vi "OE2011&OE2021_Configure Auto Phase And Filter.vi"(7 "OE2011&OE2021_\nAuto Phase And Filter":T1={"Auto Phase"=FALSE, "Auto Filter"=FALSE, "Demodulator"=1} {"Demodulator" items=["Demod1"=1, "Demod2"=2, "Demod3"=3, "Demod4"=4, "Demod5"=5, "Demod6"=6, "Demod7"=7, "Demod8"=8]}, 8 "Error in (no error)":errorcluster caption="error out（no error）", 9 "Remote Mode":u16(ring) items=["USB", "RS232", "GPIB", "Ethernet"], 10 "Connection ID in":refnum<k5>, 11 "VISA resource name":refnum<visa-resource-name>) -> (0 "Error out":errorcluster caption="error out", 1 "Output String":string, 2 "Connection ID out":refnum<k5>, 3 "VISA resource  out":refnum<visa-resource-name>)   [LabVIEW 2011]
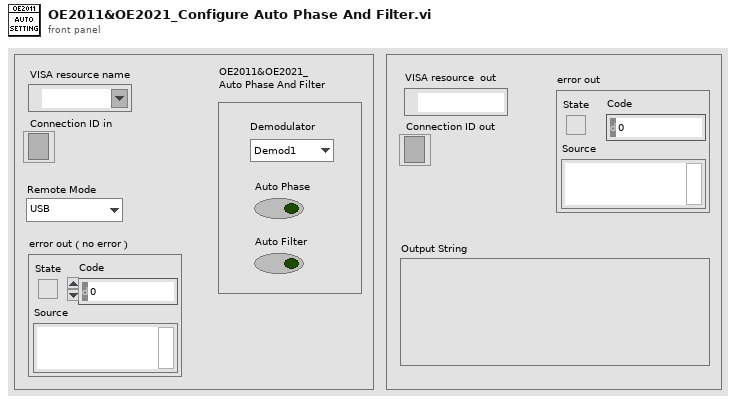
[diagram p1: front panel]
types:
  T1 = cluster{"Auto Phase":bool, "Auto Filter":bool, "Demodulator":u16}
  T2 = enum16{"ISRC", "IGND", "ICPL", "ILIN", "PHAS", "FMOD", "RSLP", "FREQ", "SWPT", "SLLM", "SULM", "SSLL", "SSLG", "STLM", "SWRM", "IRNG", "SENS", "RMOD", "OFLT", "OFSL", "SYNC", "DMOD", "HARM", "DARB", "SWVT", "SLVL", "SVLL", "SVUL", "SVSL", "SVSG", "SVTM", "SVRM", "RALL", "SNAP", "OUTP", "OAUX", "COUT", "CAUX", "COFP", "CEXP", "FPOP", "OEXP", "*IDN", "*RST", "OVLD", "INOV", "GNOV", "*PLL", "SSET", "RSET", "AGAN", "APHS", "ARSV", "ASCL", "EQCD", "EQCS", "SPED", "SRAT", "SLEN", "SSLE", "STRG", "SPRM", "STRD", "PAUS", "REST", "SPTS", "TRCA", "TEMP", "RSTU", "IHNZ", "DEQU", "SADD", "ARNG", "CSPE", "ISRCD", "IGNDD", "ICPLD", "ILIND", "PHASD", "FMODD", "RSLPD", "FREQD", "SWPTD", "SLLMD", "SULMD", "SSLLD", "SSLGD", "STLMD", "SWRMD", "SENSD", "RMODD", "OFLTD", "OFSLD", "SYNCD", "HARMD", "EQCDD", "EQCSD", "SNAPD", "OUTPD", "SWVTD", "SLVLD", "SVLLD", "SVULD", "SVSLD", "SVSGD", "SVTMD", "SVRMD", "SVDCD", "ARSVD", "AGAND", "APHSD", "ASCLD", "FPOPD", "CAUXD", "OEXPD", "SPEDD", "SRATD", "SLEND", "SSLED", "STRGD", "SPRMD", "STRDD", "PAUSD", "RESTD", "SPTSD", "TRCAD", "*IDND", "*RSTD", "INOVD", "GNOVD", "*PLLD", "SSETD", "RSETD"}
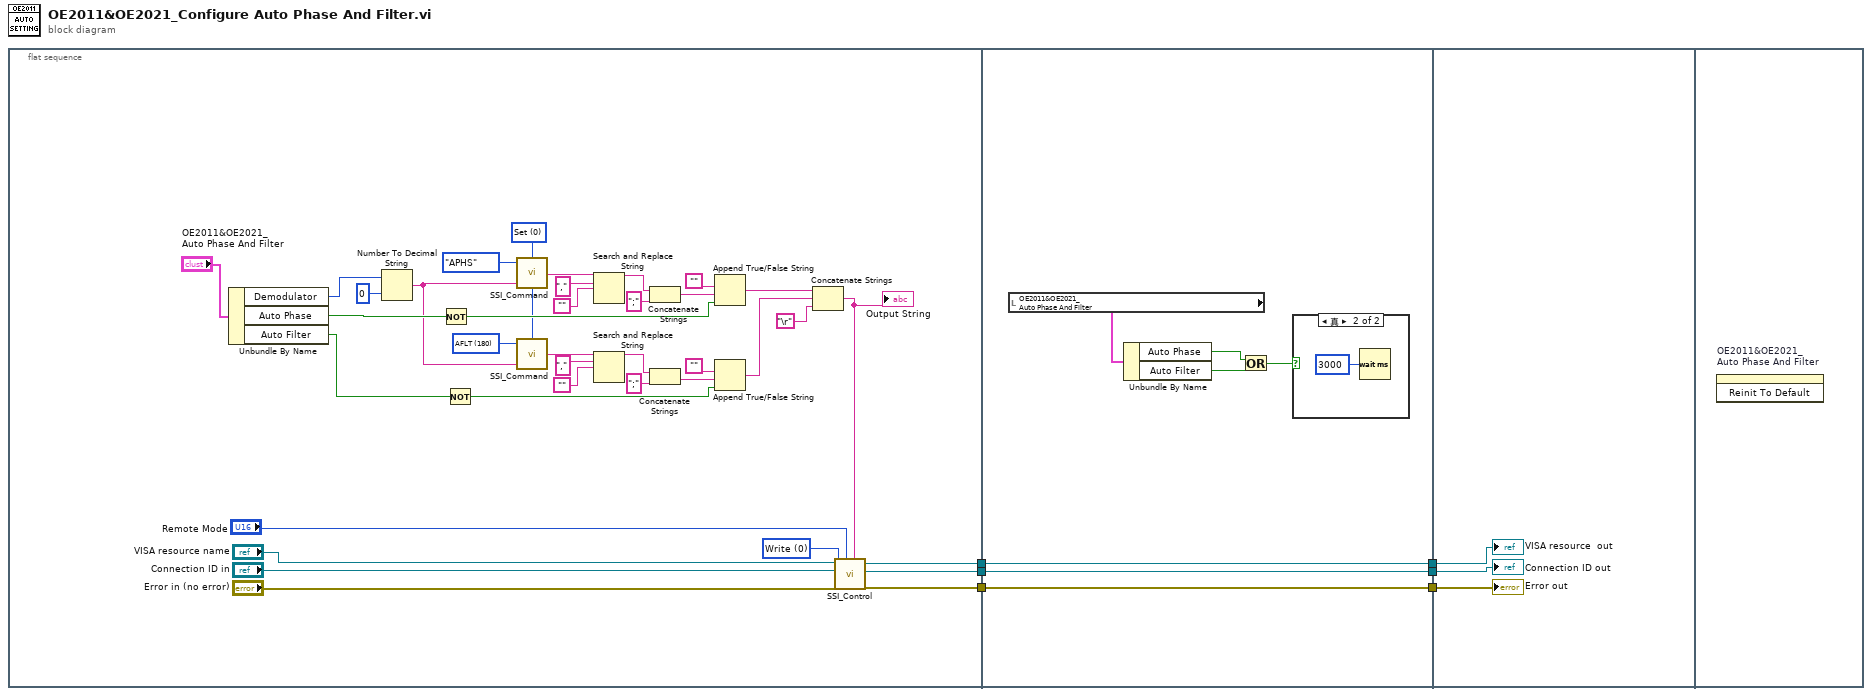
[diagram p0: block diagram]
diagram:
  n1 = flat-sequence {
    tunnel: [w39] -> w6
    tunnel: [w38] -> w5
    tunnel: [w37] -> w4
    tunnel: w6 -> [w50]
    tunnel: w5 -> [w49]
    tunnel: w4 -> [w48]
    tunnel: [w50] -> w3
    tunnel: [w49] -> w2
    tunnel: [w48] -> w1
    tunnel: w3 -> [w53]
    tunnel: w2 -> [w54]
    tunnel: w1 -> [w52]
    frame #0 {
      w13 = u16 0 items=["Set", "Query"] ("Opera")
      w18 = u16 180 items=["ISRC", "IGND", "ICPL", "ILIN", "PHAS", "FMOD", "RSLP", "FREQ", "SWPT", "SLLM", "SULM", "SSLL", "SSLG", "STLM", "SWRM", "IRNG", "SENS", "RMOD", "OFLT", "OFSL", "SYNC", "DMOD", "HARM", "DARB", "SWVT", "SLVL", "SVLL", "SVUL", "SVSL", "SVSG", "SVTM", "SVRM", "RALL", "SNAP", "OUTP", "OAUX", "COUT", "CAUX", "COFP", "CEXP", "FPOP", "OEXP", "*IDN", "*RST", "OVLD", "INOV", "GNOV", "*PLL", "SSET", "RSET", "AGAN", "APHS", "ARSV", "ASCL", "EQCD", "EQCS", "SPED", "SRAT", "SLEN", "SSLE", "STRG", "SPRM", "STRD", "PAUS", "REST", "SPTS", "TRCA", "TEMP", "RSTU", "INHZ", "DEQU", "SADD", "ARNG", "CSPE", "ISRCD", "IGNDD", "ICPLD", "ILIND", "PHASD", "FMODD", "RSLPD", "FREQD", "SWPTD", "SLLMD", "SULMD", "SSLLD", "SSLGD", "STLMD", "SWRMD", "SENSD", "RMODD", "OFLTD", "OFSLD", "SYNCD", "HARMD", "EQCDD", "EQCSD", "SNAPD", "OUTPD", "SWVTD", "SLVLD", "SVLLD", "SVULD", "SVSLD", "SVSGD", "SVTMD", "SVRMD", "SVDCD", "ARSVD", "AGAND", "APHSD", "ASCLD", "FPOPD", "CAUXD", "OEXPD", "SPEDD", "SRATD", "SLEND", "SSLED", "STRGD", "SPRMD", "STRDD", "PAUSD", "RESTD", "SPTSD", "TRCAD", "*IDND", "*RSTD", "INOVD", "GNOVD", "*PLLD", "SSETD", "RSETD", "RALLD", "NIPA", "NSMA", "NGWA", "NMAC", "NMOD", "TRIG", "TRCB", "INHZD", "ISAMD", "IRAGD", "RRAGD", "SOFFD", "DMODD", "COUTD", "COFPD", "CEXPD", "ARNGD", "OAUXD", "TRIM", "SUITD", "SNHZD", "AOFSD", "RSRC", "FEXT", "FINT", "DSRC", "DARF", "DEAF", "DREF", "SSRC", "STTL", "SIGO", "SLVL", "SOFF", "SPHS", "TPHS", "SMOD", "MARF", "AMSR", "AMDP", "FMSR", "FMDV", "PMSR", "PMDV", "CHDC", "AUXV", "AFLT", "AOFP"] ("Command Type")
      w40 = u16 0 items=["Write", "Read"] ("Control")
      n2 = Unbundle By Name("OE2011&OE2021_\nAuto Phase And Filter") -> ("Demodulator"=w15:u16, "Auto Phase"=w20:bool, "Auto Filter"=w17:bool)
      n3 = Number To Decimal String(number=w15, width (-)=i16 0 ("宽度(-)")) -> (decimal integer string=w14:string)
      n4 = Not(x=w20) -> (.not. x?=w19:bool)
      n5 = Not(x=w17) -> (.not. x?=w12:bool)
      n6 = call "SSI_Command.vi"("Opera"=w13, "Paramter"=w14, "Command Type"=T2."APHS") -> ("Output string"=w23:string)  [unwired: 1 in]
      n7 = call "SSI_Command.vi"("Opera"=w13, "Paramter"=w14, "Command Type"=w18) -> ("Output string"=w22:string)  [unwired: 1 in]
      n8 = Search and Replace String(input string=w23, search string="," ("搜索字符串"), replace string="") -> (result string=w29:string)  [unwired: 5 in, 3 out]
      n9 = Search and Replace String(input string=w22, search string="," ("搜索字符串"), replace string="") -> (result string=w26:string)  [unwired: 5 in, 3 out]
      n10 = Concatenate Strings(w29, ";") -> (w25:string)
      n11 = Concatenate Strings(w26, ";") -> (w24:string)
      n12 = Append True/False String(1:w19, 2:w25, 3:"") -> (0:w8:string)  [unwired: 1 in]
      n13 = Append True/False String(1:w12, 2:w24, 3:"") -> (0:w7:string)  [unwired: 1 in]
      n14 = Concatenate Strings(w8, w7, "\r") -> (w10:string)
      "Output String" <- w10
      n15 = call "SSI_Control.vi"("Write Buffer"=w10, "Remote Mode"="Remote Mode", "Error in (no error)"="Error in (no error)", "Control"=w40, "Connection ID in"="Connection ID in", "VISA resource name"="VISA resource name") -> ("Error out"=w37:errorcluster, "Connection ID out"=w39:refnum<k5>, "VISA resource  out"=w38:refnum<visa-resource-name>)  [unwired: 2 in, 1 out]
    }
    frame #1 {
      n16 = local read "OE2011&OE2021_\nAuto Phase And Filter"() -> (w47:T1)
      n17 = Unbundle By Name(w47) -> ("Auto Phase"=w46:bool, "Auto Filter"=w45:bool)
      n18 = Or(x=w46, y=w45) -> (x .or. y?=w44:bool)
      n19 = case shown="真" w44 {
        frame False {
        }
        frame True {
          n20 = Wait (ms)(milliseconds to wait=u32 3000 ("等待时间（毫秒）")) -> ()  [unwired: 1 out]
        }
      }
    }
    frame #2 {
      "Error out" <- w52
      "Connection ID out" <- w53
      "VISA resource  out" <- w54
    }
    frame #3 {
      n21 = invoke on="OE2011&OE2021_\nAuto Phase And Filter" class="Clust (严格)" method="Reinit To Default"() -> ()  [unwired: 3 in, 3 out]
    }
  }
